vi "CloseXL_App.vi"(8 "error in (no error)":errorcluster, 11 "Refnum Cluster In":T1) -> (0 "error out":errorcluster)   [LabVIEW 2015]
doc: "This VI closes the XL application opened by OpenXL_App.vi."
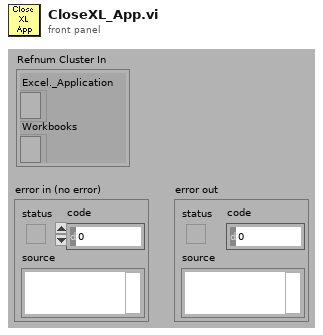
[diagram p1: front panel]
types:
  T1 = cluster{"Excel._Application":refnum<k7>, "Workbooks":refnum<k7>}
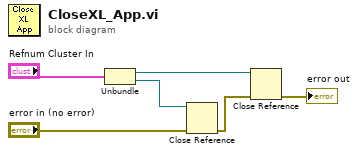
[diagram p0: block diagram]
diagram:
  n1 = Unbundle("Refnum Cluster In") -> ("Excel._Application"=w3:refnum<k7>, "Workbooks"=w2:refnum<k7>)
  n2 = Close Reference(reference=w2, error in (no error)="error in (no error)") -> (error out=w4:errorcluster)
  n3 = Close Reference(reference=w3, error in (no error)=w4) -> (error out=→"error out":errorcluster)
